vi "Read URLs from Variant.vi"(3 "Error In":errorcluster, 4 "URL Section Data":variant, 5 "URL Prefix":string) -> (0 "Error Out":errorcluster, 1 "URLs":string[](array[string]), 2 "Found?":bool)   [LabVIEW 2013, in "CS++DCPwr.lvlib" / "CS++DCPwr.lvclass"]
doc: "Read rray of URL strings corresponding to specified Prefix from variant containing URL section data."
uses:
  CS++DCPwr.lvclass
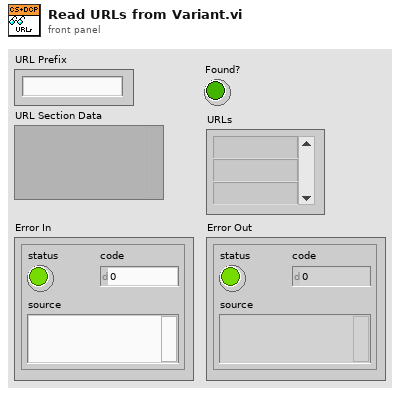
[diagram p1: front panel]
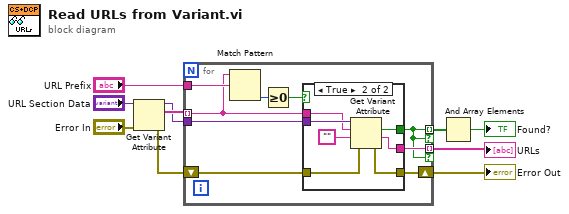
[diagram p0: block diagram]
diagram:
  n1 = Get Variant Attribute(Variant="URL Section Data", error in="Error In") -> (duplicate Variant=w7:variant, names=w8:string[], error out=w9:errorcluster)  [unwired: 2 in, 1 out]
  n2 = for {
    tunnel: [w11] -> w10 mode=indexing if=w11
    tunnel: w7 -> [w17]
    shift-right: [w19] -> w3
    shift-left: w9 -> [w18]
    tunnel: w8 -> [w15] mode=indexing
    tunnel: "URL Prefix" -> [w16]
    tunnel: [w12] -> w1 mode=indexing if=w11
    n3 = Match Pattern(string=w15, regular expression=w16) -> (offset past match=w14:i32)  [unwired: 1 in, 3 out]
    n4 = Greater Or Equal To 0?(x=w14) -> (x >= 0?=w13:bool)
    n5 = case shown="True" w13 {
      tunnel: [_ w26] -> w11
      tunnel: [w20 w25] -> w19
      tunnel: w18 -> [w20 w24]
      tunnel: w17 -> [_ w23]
      tunnel: w15 -> [_ w22]
      tunnel: [_ w21] -> w12
      frame False {
      }
      frame True {
        n6 = Get Variant Attribute(Variant=w23, name=w22, default value (empty Variant)="", error in=w24) -> (found=w26:bool, value=w21:string, error out=w25:errorcluster)  [unwired: 1 out]
      }
    }
  }
  "Error Out" <- w3
  "URLs" <- w1
  n7 = And Array Elements(Boolean array=w10) -> (logical AND=→"Found?":bool)
